vi "Test Window Position Size.vi"() -> ()   [LabVIEW 2012]
panel:
  in  "Boolean":bool
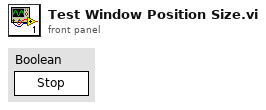
[diagram p1: front panel]
types:
  T1 = enum32{"Invalid", "Standard", "Closed", "Hidden", "Minimized", "Maximized"}
  T2 = typedef "LVAllMonitorsDisplayTypeDef.ctl" = cluster{"Bounds":cluster{"Left":i16, "Top":i16, "Right":i16, "Bottom":i16}, "Depth":i16}[]
  T3 = cluster{"Bounds":cluster{"Left":i16, "Top":i16, "Right":i16, "Bottom":i16}, "Depth":i16}
  T4 = cluster{"Left":i16, "Top":i16, "Right":i16, "Bottom":i16}
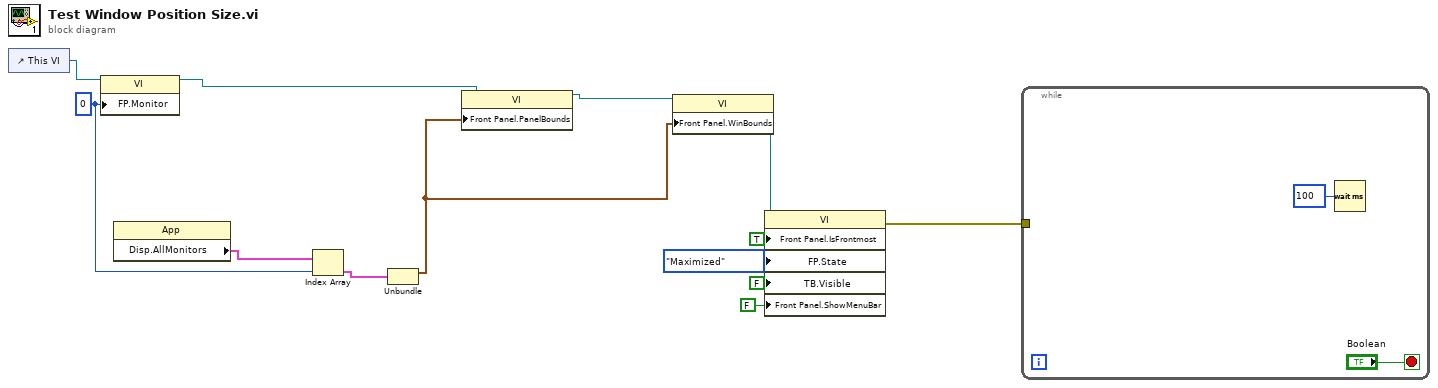
[diagram p0: block diagram]
diagram:
  w11 = u16 0 ("Front Panel Window:Monitor")
  n1 = control-ref of="This VI"() -> (w13:refnum<vi>)
  n2 = property class="VI"(reference=w13, "FP.Monitor"=w11) -> (reference out=w9:refnum<vi>)  [unwired: 1 in, 1 out]
  n3 = property class="App"() -> ("Disp.AllMonitors"=w12:T2)  [unwired: 2 in, 2 out]
  n4 = Index Array(array=w12, index=w11) -> (element=w10:T3)
  n5 = Unbundle(w10) -> ("Bounds"=w7:T4)  [unwired: 1 out]
  n6 = property class="VI"(reference=w9, "Front Panel.PanelBounds"=w7) -> (reference out=w8:refnum<vi>)  [unwired: 1 in, 1 out]
  n7 = property class="VI"(reference=w8, "Front Panel.WinBounds"=w7) -> (reference out=w6:refnum<vi>)  [unwired: 1 in, 1 out]
  n8 = property class="VI"(reference=w6, "Front Panel.IsFrontmost"=TRUE ("Front Panel Window:Is Frontmost"), "FP.State"=T1."Maximized" ("Front Panel Window:State"), "TB.Visible"=FALSE ("Tool Bar:Visible"), "Front Panel.ShowMenuBar"=FALSE ("Front Panel Window:Show Menu Bar")) -> (error out=w3:errorcluster)  [unwired: 1 in, 1 out]
  n9 = while {
    tunnel: w3 -> [_]
    stop <- "Boolean" stop-if-true
    n10 = Wait (ms)(milliseconds to wait=u32 100) -> ()  [unwired: 1 out]
  }
